vi "Type Mask.vi"(7 "Address":string, 8 "Error In":errorcluster) -> (0 "Error Out":errorcluster)   [LabVIEW 2018, in "Tests.lvlib" / "Known Host.lvlib"]
uses:
  Known Host.lvlib
  <vilib>/addons/_JKI Toolkits/Caraya/classes/Test/Test.lvclass
  <vilib>/addons/_JKI Toolkits/Caraya/classes/Assert/Assert.lvclass
  src/Toolkit/Known Host/Known Host.lvclass
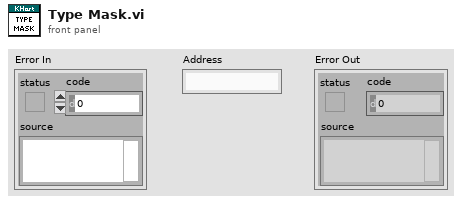
[diagram p1: front panel]
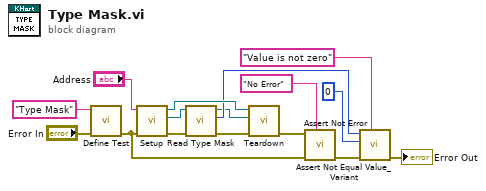
[diagram p0: block diagram]
diagram:
  n1 = call <vilib>:"Define Test.vi"("error in (no error)"="Error In", "Label (VI Title)"="Type Mask") -> ("error out"=w12:errorcluster)  [unwired: 9 in]
  n2 = call "Setup.vi"("Error In"=w12, "Address"="Address") -> ("Error Out"=w5:errorcluster, "Known Host"=w2:refnum<class "Known Host.lvclass">, "Known Hosts"=w10:refnum<class "Known Hosts.lvclass">)  [unwired: 7 in]
  n3 = call "Read Type Mask.vi"("Error In"=w5, "Known Host In"=w2) -> ("Error Out"=w4:errorcluster, "Type Mask"=w3:i32, "Known Host Out"=w1:refnum<class "Known Host.lvclass">)  [unwired: 7 in]
  n4 = call "Teardown.vi"("Error In"=w4, "Known Host"=w1, "Known Hosts"=w10) -> ("Error Out"=w9:errorcluster)  [unwired: 8 in]
  n5 = call <vilib>:"Assert Not Error.vi"("Label"="No Error", "error in (no error)"=w12, "Not Error?"=w9) -> ("error out"=w13:errorcluster)  [unwired: 8 in]
  n6 = call <vilib>:"Assert Not Equal Value_Variant.vi"("Label"="Value is not zero", "error in (no error)"=w13, "Y"=0 ("Magic"), "X"=w3) -> ("error out"=→"Error Out":errorcluster)  [unwired: 7 in]
